vi "stop_tasks.vi"(8 "error in (no error)":errorcluster, 11 "Experiment in":refnum<class "Experiment.lvclass">) -> (0 "error out":errorcluster, 3 "Experiment out":refnum<class "Experiment.lvclass">)   [LabVIEW 2013, in "Experiment.lvclass"]
uses:
  Experiment.lvclass
  Experiment.lvclass/Experiment.ctl
  Counter/Counter.lvclass
  Analog_output/Analog_Output.lvclass
  HSDIO/HSDIO.lvclass
  DAQmx_pulse_out/DAQmx_pulse_out.lvclass
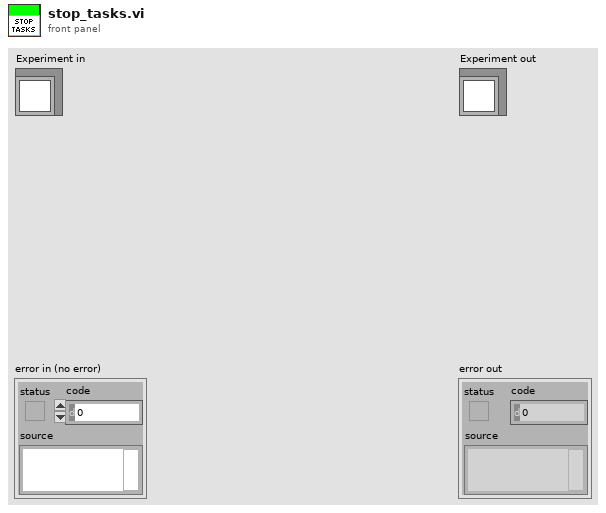
[diagram p1: front panel]
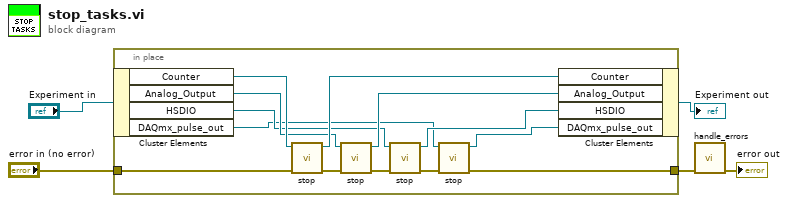
[diagram p0: block diagram]
diagram:
  n1 = in-place {
    in-place-border: "error in (no error)" -> [w10]
    in-place-border: [w6] -> w1
    n2 = in-place-cluster #1("Experiment in") -> ("Counter"=w18:refnum<class "Counter.lvclass">, "Analog_Output"=w16:refnum<class "Analog_Output.lvclass">, "HSDIO"=w14:refnum<class "HSDIO.lvclass">, "DAQmx_pulse_out"=w12:refnum<class "DAQmx_pulse_out.lvclass">)
    n3 = call-dynamic "stop.vi"("error in (no error)"=w10, "Counter in"=w18) -> ("error out"=w9:errorcluster, "Counter out"=w17:refnum<class "Counter.lvclass">)  [unwired: 8 in]
    n4 = call-dynamic "stop.vi"("error in (no error)"=w9, "Analog_Output in"=w16) -> ("error out"=w8:errorcluster, "Analog_Output out"=w15:refnum<class "Analog_Output.lvclass">)  [unwired: 8 in]
    n5 = call-dynamic "stop.vi"("error in (no error)"=w8, "HSDIO in"=w14) -> ("error out"=w7:errorcluster, "HSDIO out"=w13:refnum<class "HSDIO.lvclass">)  [unwired: 8 in]
    n6 = call-dynamic "stop.vi"("error in (no error)"=w7, "DAQmx_pulse_out in"=w12) -> ("error out"=w6:errorcluster, "DAQmx_pulse_out out"=w11:refnum<class "DAQmx_pulse_out.lvclass">)  [unwired: 8 in]
    n7 = in-place-cluster #1("Counter"=w17, "Analog_Output"=w15, "HSDIO"=w13, "DAQmx_pulse_out"=w11) -> (→"Experiment out":refnum<class "Experiment.lvclass">)
  }
  n8 = call "handle_errors.vi"("error in (no error)"=w1) -> ("error out"=→"error out":errorcluster)  [unwired: 14 in]
